vi "fuzzy theta calculation sum method.vi"(7 "Theta In":dbl, 8 "obstcls Y":dbl[](array[numeric]), 9 "obstcls X":dbl[](array[numeric]), 10 "Y ref":dbl=1980.0, 11 "X ref":dbl) -> (2 "Theta Out":dbl)   [LabVIEW 2011]
panel:
  out "closeness to obstcls":dbl
  out "sum y":dbl
  out "sum x":dbl
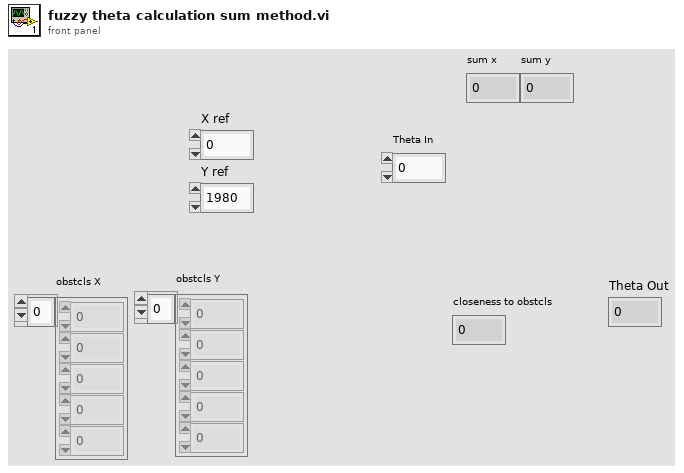
[diagram p1: front panel]
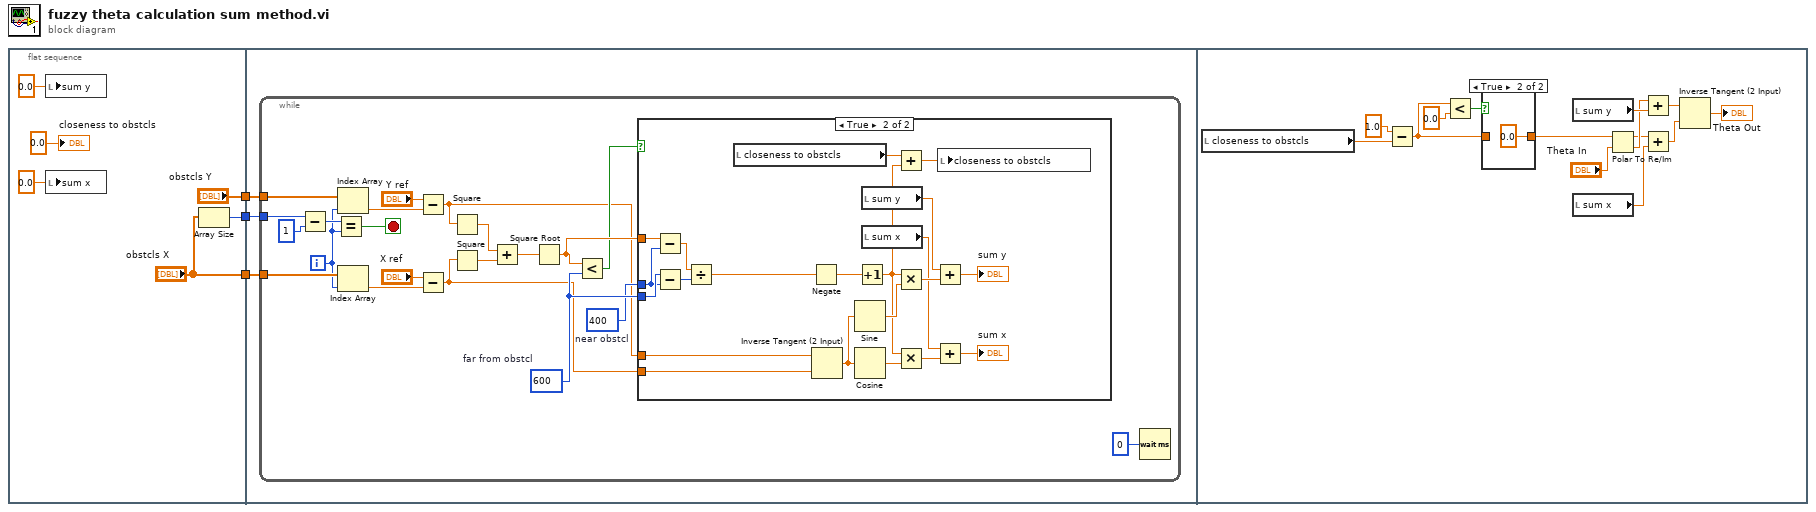
[diagram p0: block diagram]
diagram:
  n1 = flat-sequence {
    tunnel: ["obstcls X"] -> w3
    tunnel: ["obstcls Y"] -> w2
    tunnel: [w7] -> w1
    tunnel: w3 -> [w12]
    tunnel: w2 -> [w11]
    tunnel: w1 -> [w10]
    frame #0 {
      n2 = local write "sum y"(0.0 ("sum y")) -> ()
      n3 = local write "sum x"(0.0 ("sum y")) -> ()
      n4 = Array Size(array="obstcls X") -> (size(s)=w7:i32)
      "closeness to obstcls" <- 0.0 ("closeness")
    }
    frame #1 {
      n5 = while {
        tunnel: w12 -> [w18]
        tunnel: w11 -> [w17]
        tunnel: w10 -> [w16]
        i -> [w13]
        stop <- w23 stop-if-true
        w27 = 400  # near obstcl
        w28 = 600  # far from obstcl
        n6 = Subtract(x=w16, y=1) -> (x-y=w14:i32)
        n7 = Equal?(x=w14, y=w13) -> (x = y?=w23:bool)
        n8 = Index Array(array=w17, index=w13) -> (element=w21:dbl)
        n9 = Index Array(array=w18, index=w13) -> (element=w22:dbl)
        n10 = Subtract(x="Y ref", y=w21) -> (x-y=w20:dbl)
        n11 = Subtract(x="X ref", y=w22) -> (x-y=w19:dbl)
        n12 = Square(x=w20) -> (x^2=w29:dbl)
        n13 = Square(x=w19) -> (x^2=w33:dbl)
        n14 = Add(x=w29, y=w33) -> (x+y=w30:dbl)
        n15 = Square Root(x=w30) -> (sqrt(x)=w32:dbl)
        n16 = Less?(x=w32, y=w28) -> (x < y?=w31:bool)
        n17 = case shown="True" w31 {
          tunnel: w27 -> [_ w52]
          tunnel: w32 -> [_ w54]
          tunnel: w28 -> [_ w53]
          tunnel: w20 -> [_ w42]
          tunnel: w19 -> [_ w41]
          frame False {
          }
          frame True {
            n18 = Subtract(x=w54, y=w52) -> (x-y=w49:dbl)
            n19 = Subtract(x=w53, y=w52) -> (x-y=w51:i32)
            n20 = Divide(x=w49, y=w51) -> (x/y=w48:dbl)
            n21 = local read "closeness to obstcls"() -> (w36:dbl)
            n22 = Negate(x=w48) -> (-x=w50:dbl)
            n23 = Inverse Tangent (2 Input)(1:w41, 2:w42) -> (0:w39:dbl)
            n24 = Sine(x=w39) -> (sin(x)=w40:dbl)
            n25 = Cosine(x=w39) -> (cos(x)=w38:dbl)
            n26 = Increment(x=w50) -> (x+1=w35:dbl)
            n27 = local read "sum y"() -> (w37:dbl)
            n28 = local read "sum x"() -> (w43:dbl)
            n29 = Add(x=w36, y=w35) -> (x+y=w34:dbl)
            n30 = Multiply(x=w35, y=w40) -> (x*y=w47:dbl)
            n31 = Multiply(x=w35, y=w38) -> (x*y=w46:dbl)
            n32 = Add(x=w37, y=w47) -> (x+y=→"sum y":dbl)
            n33 = Add(x=w43, y=w46) -> (x+y=→"sum x":dbl)
            n34 = local write "closeness to obstcls"(w34) -> ()
          }
        }
        n35 = Wait (ms)(milliseconds to wait=u32 0) -> ()  [unwired: 1 out]
      }
    }
    frame #2 {
      n36 = local read "closeness to obstcls"() -> (w59:dbl)
      n37 = Subtract(x=1.0 ("r"), y=w59) -> (x-y=w56:dbl)
      n38 = Less?(x=w56, y=0.0) -> (x < y?=w55:bool)
      n39 = case shown="True" w55 {
        tunnel: [w69 0.0 ("y")] -> w57
        tunnel: w56 -> [w69 _]
        frame False {
        }
        frame True {
        }
      }
      n40 = local read "sum y"() -> (w67:dbl)
      n41 = local read "sum x"() -> (w66:dbl)
      n42 = Polar To Re/Im(2:"Theta In", 3:w57) -> (0:w63:dbl, 1:w62:dbl)
      n43 = Add(x=w63, y=w67) -> (x+y=w65:dbl)
      n44 = Add(x=w62, y=w66) -> (x+y=w64:dbl)
      n45 = Inverse Tangent (2 Input)(1:w64, 2:w65) -> (0:→"Theta Out":dbl)
    }
  }
